vi "ThirdStageRelease.vi"(10 "In":bool, 11 "Out":bool) -> ()   [LabVIEW 2018]
uses:
  <vilib>/Rock Robotics/WPI/Solenoid/WPI_SolenoidValue.ctl
  <vilib>/Rock Robotics/WPI/Solenoid/WPI_SolenoidSetEnum.vi
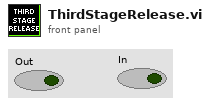
[diagram p1: front panel]
types:
  T1 = typedef "WPI_SolenoidValue.ctl" = enum16{"Off", "On", "Forward", "Reverse"}
  T2 = typedef "WPI_SolenoidDevRef.ctl" = cluster{"DevStatus":errorcluster, "Pneumatics Control Module":u8, "Forward Solenoid Channel":T3, "Reverse Solenoid Channel":T3}
  T3 = typedef "WPI_SolenoidChannel.ctl" = enum8{"Solenoid 0", "Solenoid 1", "Solenoid 2", "Solenoid 3", "Solenoid 4", "Solenoid 5", "Solenoid 6", "Solenoid 7", "Invalid"}
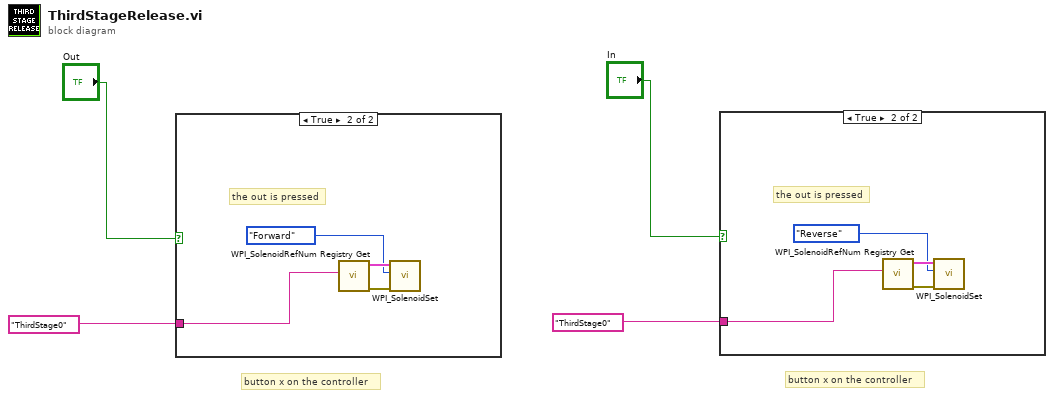
[diagram p0: block diagram]
diagram:
  # "button x on the controller"
  # "button x on the controller"
  n1 = case shown="True" "Out" {
    tunnel: "ThirdStage0" ("refnum name") -> [_ w5]
    frame False {
    }
    frame True {
      # "the out is pressed"
      n2 = call <vilib>:"WPI_SolenoidRefNum Registry Get.vi"("refnum name"=w5) -> ("error out"=w7:errorcluster, "SolenoidDevRef"=w8:T2)  [unwired: 9 in]
      n3 = call-poly <vilib>:"WPI_SolenoidSet.vi"("error in (no error)"=w7, "Value"=WPI_SolenoidValue."Forward", "SolenoidDevRef"=w8) -> ()  [unwired: 7 in, 2 out]
    }
  }
  n4 = case shown="True" "In" {
    tunnel: "ThirdStage0" ("refnum name") -> [_ w9]
    frame False {
    }
    frame True {
      # "the out is pressed"
      n5 = call <vilib>:"WPI_SolenoidRefNum Registry Get.vi"("refnum name"=w9) -> ("error out"=w11:errorcluster, "SolenoidDevRef"=w12:T2)  [unwired: 9 in]
      n6 = call-poly <vilib>:"WPI_SolenoidSet.vi"("error in (no error)"=w11, "Value"=WPI_SolenoidValue."Reverse", "SolenoidDevRef"=w12) -> ()  [unwired: 7 in, 2 out]
    }
  }
